vi "Encapsulate UDP Message.vi"(5 "source_id":u32, 8 "error in (no error)":errorcluster, 9 "type":string, 10 "Encapsulated Msg":refnum<class "Message.lvclass">, 11 "SequenceCountService":refnum<class "SequenceCountService.lvclass">) -> (0 "error out":errorcluster, 2 "UDP Payload":string)   [LabVIEW 2020, in "Vecto.lvlib"]
uses:
  Vecto.lvlib
  lv-protoc/LV-Proto/Message/Message.lvclass
  SequenceCountService/SequenceCountService.lvclass
  lv-volatus/messages/UdpPayload/Data.ctl
  SequenceCountService/SequenceCountService.lvclass/SequenceCountService.ctl
  lv-volatus/messages/UdpPayload/UdpPayload.lvlib
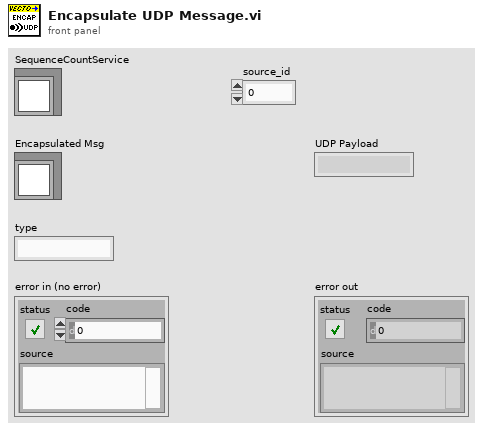
[diagram p1: front panel]
types:
  T1 = typedef "UdpPayload.lvlib/Data.ctl" = cluster{"source_id":u32, "sequence":u32, "timestamp":i64, "type":string, "payload":u8[]}
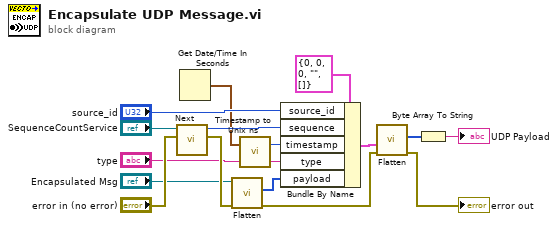
[diagram p0: block diagram]
diagram:
  n1 = call "Next.vi"("error in (no error)"="error in (no error)", "SequenceCountService in"="SequenceCountService") -> ("error out"=w15:errorcluster, "Sequence"=w8:u32)  [unwired: 8 in]
  n2 = Get Date/Time In Seconds() -> (seconds since 1Jan1904=w1:timestamp)
  n3 = call-dynamic "Flatten.vi"("error in (no error)"=w15, "Message in"="Encapsulated Msg") -> ("error out"=w4:errorcluster, "Buffer"=w10:u8[])  [unwired: 7 in, 1 out]
  n4 = call "Timestamp to Unix ns.vi"("Time Stamp"=w1) -> ("unix ns"=w2:i64)  [unwired: 2 in]
  n5 = Bundle By Name(cluster=T1 {"source_id"=0, "sequence"=0, "timestamp"=0, "type"="", "payload"=[]} ("UdpPayload"), "source_id"="source_id", "sequence"=w8, "timestamp"=w2, "type"="type", "payload"=w10) -> (w7:T1)
  n6 = call "Flatten.vi"("error in"=w4, "Data"=w7) -> ("error out"=→"error out":errorcluster, "Buffer"=w6:u8[])  [unwired: 8 in]
  n7 = Byte Array To String(unsigned byte array=w6) -> (string=→"UDP Payload":string)
